vi "Bytes at port eq to 0 or less y.vi"(0 "y":u32=4, 1 "Bytes at Port":u32) -> (4 "Bytes at port = 0 or less y":bool, 7 "Bytes at Port out":u32)   [LabVIEW 2012]
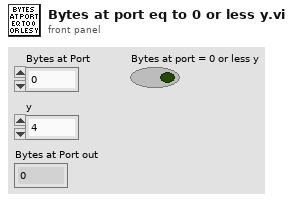
[diagram p1: front panel]
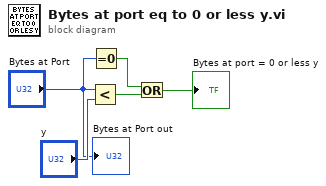
[diagram p0: block diagram]
diagram:
  n1 = Less?(x="Bytes at Port", y="y") -> (x < y?=w4:bool)
  n2 = Equal To 0?(x="Bytes at Port") -> (x = 0?=w3:bool)
  n3 = Or(x=w3, y=w4) -> (x .or. y?=→"Bytes at port = 0 or less y":bool)
  "Bytes at Port out" <- "Bytes at Port"
